vi "XYZ Stage-StatusMonitor.vi"(0 "VISA resource name":refnum<visa-resource-name>="COM1", 1 "Send command? (T)":bool=TRUE, 5 "string to write":string="*IDN?\r\n", 11 "Error In":errorcluster, 12 "Read response? (T)":bool=TRUE) -> (4 "VISA resource name out":refnum<visa-resource-name>, 6 "read string":string, 8 "Empty response string":bool, 10 "bytes read":u32, 15 "Error Out":errorcluster)   [LabVIEW 2020]
uses:
  <vilib>/Instr/_visa.llb/VISA Configure Serial Port (Instr).vi
panel:
  in  "delay after read (ms)":u32=50
  in  "delay before read (ms)":u32=60
  in  "flow control":u16(ring) items=["None"=0, "XON/XOFF"=1, "RTS/CTS"=2, "DTR/DSR"=4]
  in  "stop bits":u16(ring)=10 items=["1.0"=10, "1.5"=15, "2.0"=20]
  in  "parity":u16(ring) items=["None", "Odd", "Even", "Mark", "Space"]
  in  "data bits":u16=8 min=5 max=8 step=1
  in  "baud rate":u32=9600
  # "<---Do not set less that 60ms. Below 50ms all sort of weird things start happening."
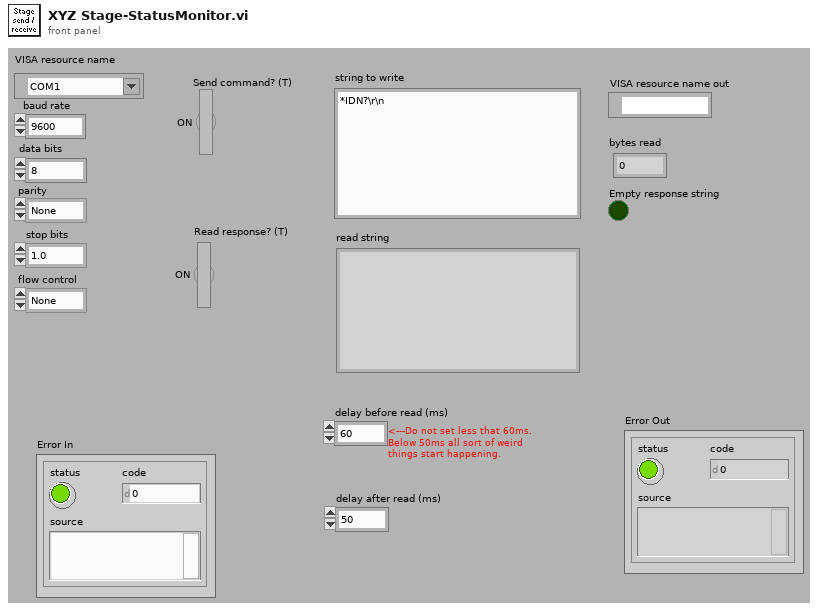
[diagram p1: front panel]
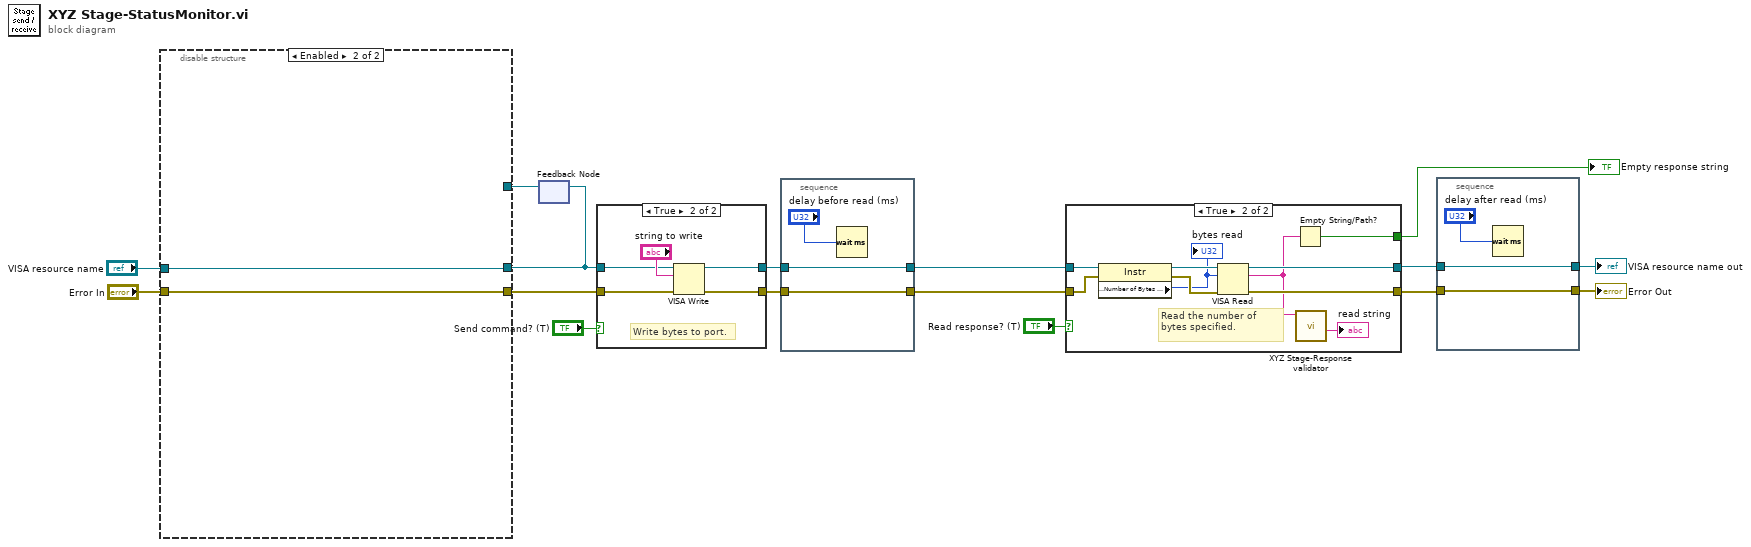
[diagram p0: block diagram]
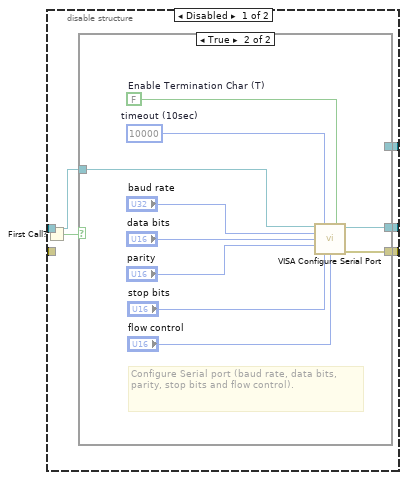
[diagram p2: hidden frame]
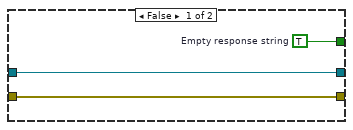
[diagram p5: hidden frame]
diagram:
  n1 = feedback #1() -> (w9:refnum<visa-resource-name>)  [unwired: 1 in]
  n2 = disable-structure "Diagram Disable Structure" shown="Enabled" {
    disable-tunnel: [w21 w33] -> w15
    disable-tunnel: w9 -> [w19 _]
    disable-tunnel: [w18 w34] -> w8
    disable-tunnel: "VISA resource name" -> [w17 w34]
    disable-tunnel: "Error In" -> [_ w33]
    frame Disabled {
      n3 = First Call?() -> (First Call?: T/F=w20:bool)
      n4 = case shown="True" w20 {
        tunnel: [_ w31] -> w21
        tunnel: [w22 w30] -> w18
        tunnel: w19 -> [w22 _]
        tunnel: w17 -> [_ w23]
        frame False {
        }
        frame True {
          w27 = FALSE  # Enable Termination Char (T)
          w28 = u32 10000  # timeout (10sec)
          # "Configure Serial port (baud rate, data bits, parity, stop bits and flow control)."
          n5 = call-poly "VISA Configure Serial Port"("VISA resource name"=w23, "timeout (10sec)"=w28, "Enable Termination\nChar (T)"=w27, "baud rate (9600)"="baud rate", "data bits (8)"="data bits", "parity (0:none)"="parity", "stop bits (10: 1 bit)"="stop bits", "flow control (0:none)"="flow control") -> ("VISA resource name out"=w30:refnum<visa-resource-name>, "error out"=w31:errorcluster)  [unwired: 1 in, 5 out]
        }
      }
    }
    frame Enabled {
    }
  }
  n6 = feedback-in #1(w8) -> ()
  n7 = case shown="True" "Send command? (T)" {
    tunnel: [w36 w41] -> w13
    tunnel: w8 -> [w35 w39]
    tunnel: w15 -> [w36 w38]
    tunnel: [w35 w37] -> w11
    frame False {
    }
    frame True {
      # "Write bytes to port."
      n8 = VISA Write(VISA resource name=w39, write buffer="string to write", error in (no error)=w38) -> (VISA resource name out=w37:refnum<visa-resource-name>, error out=w41:errorcluster)  [unwired: 1 out]
    }
  }
  n9 = stacked-sequence {
    tunnel: w13 -> [w44]
    tunnel: [w44] -> w12
    tunnel: w11 -> [w43]
    tunnel: [w43] -> w10
    frame #0 {
      n10 = Wait (ms)(milliseconds to wait="delay before read (ms)") -> ()  [unwired: 1 out]
    }
  }
  n11 = case shown="True" "Read response? (T)" {
    tunnel: w12 -> [w47 w53]
    tunnel: [w47 w57] -> w4
    tunnel: [w46 w56] -> w5
    tunnel: w10 -> [w46 w55]
    tunnel: [w45 w50] -> w1
    frame False {
      w45 = TRUE  # Empty response string
    }
    frame True {
      # "Read the number of bytes specified."
      n12 = property class="Instr"(reference=w55, error in=w53) -> (reference out=w54:refnum<visa-resource-name>, error out=w52:errorcluster, "Serial Settings:Number of Bytes at Serial Port"=w51:u32)
      "bytes read" <- w51
      n13 = VISA Read(VISA resource name=w54, byte count=w51, error in (no error)=w52) -> (VISA resource name out=w56:refnum<visa-resource-name>, read buffer=w49:string, error out=w57:errorcluster)  [unwired: 1 out]
      n14 = Empty String/Path?(string/path=w49) -> (empty?=w50:bool)
      n15 = call "XYZ Stage-Response validator.vi"("response string"=w49) -> ("Filtered response"=→"read string":string)  [unwired: 9 in, 1 out]
    }
  }
  "Empty response string" <- w1
  n16 = stacked-sequence {
    tunnel: w4 -> [w60]
    tunnel: [w60] -> w3
    tunnel: w5 -> [w59]
    tunnel: [w59] -> w2
    frame #0 {
      n17 = Wait (ms)(milliseconds to wait="delay after read (ms)") -> ()  [unwired: 1 out]
    }
  }
  "VISA resource name out" <- w2
  "Error Out" <- w3
